vi "Write Characteristics file reference.vi"(8 "error in (no error)":errorcluster, 10 "Characteristics file reference":refnum<k34>, 11 "Analysis params in":refnum<class "CV-Analysis.lvclass">) -> (0 "error out":errorcluster, 3 "Analysis params out":refnum<class "CV-Analysis.lvclass">)   [LabVIEW 2013, in "CameraVision.lvlib" / "CV-Analysis.lvclass"]
uses:
  CV-Analysis.lvclass
  CV-Analysis.lvclass/CV-Analysis.ctl
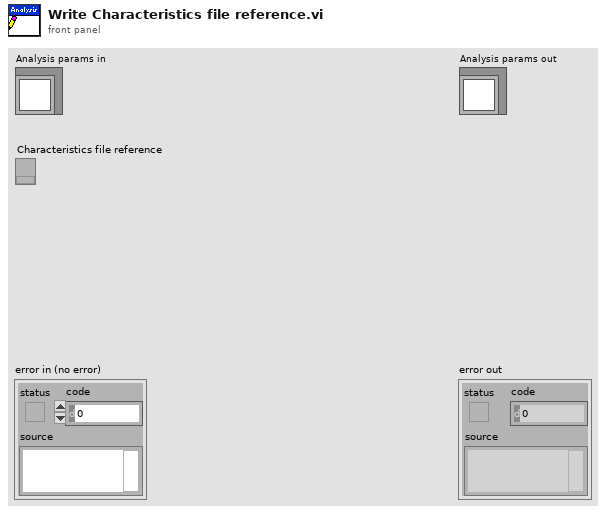
[diagram p1: front panel]
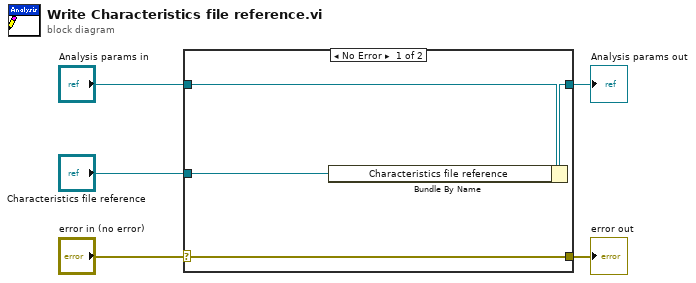
[diagram p0: block diagram]
diagram:
  n1 = case shown="No Error" "error in (no error)" {
    selector: "error in (no error)" -> [w9 w10]
    tunnel: [w9 w10] -> w4
    tunnel: [w7 w11] -> w2
    tunnel: "Analysis params in" -> [w8 w11]
    tunnel: "Characteristics file reference" -> [w6 _]
    frame No Error {
      n2 = Bundle By Name(cluster=w8, "Characteristics file reference"=w6) -> (w7:refnum<class "CV-Analysis.lvclass">)
    }
    frame Error {
    }
  }
  "error out" <- w4
  "Analysis params out" <- w2
